vi "Fluke 28x Series Software Triggered Freqency Sweep.vi"() -> ()   [LabVIEW 2015]
doc: "This example shows how to configure a frequency sweep using a software trigger."
uses:
  <instrlib>/Fluke 28x Series/Fluke 28x Series.lvlib
panel:
  in  "Stop  Frequency  (1000.0 Hz)":dbl=1000.0 format="%#.6f"
  in  "Start Frequency (100.0 Hz)":dbl=100.0 format="%#.6g"
  in  "Sweep Time (1.00 s)":dbl=1.0 format="%#.6g"
  in  "Sweep Type (0: Continuous)":u16(ring) items=["Continuous", "Triggered", "Triggered, Hold/Reset"]
  in  "Amplitude (1.0 Vpp)":dbl=1.0
  in  "Waveform Function (0: Sine)":u16(ring) items=["Sine", "Square", "Triangle", "Cosine", "DC", "Positive Ramp", "Negative Ramp", "Haversine", "Havercosine", "Sine (x)/x"]
  in  "Channel (1)":u32(ring)=1 items=["1"=1, "2"=2, "3"=3, "4"=4]
  in  "VISA resource name":refnum<visa-resource-name>
  # "(c) 2009-2014 National Instruments.  ALL RIGHTS RESERVED."
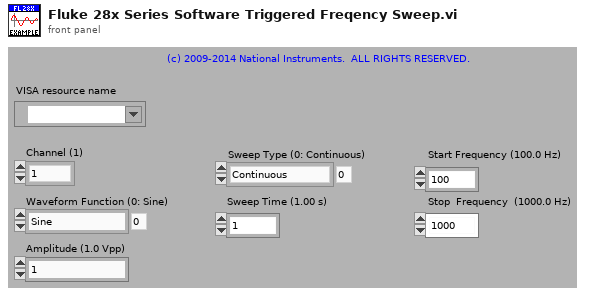
[diagram p1: front panel]
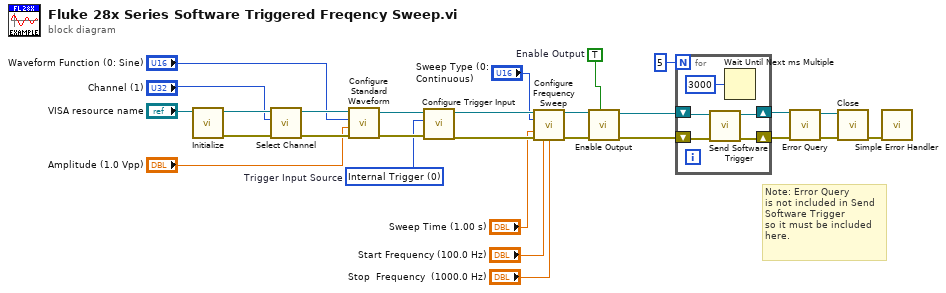
[diagram p0: block diagram]
diagram:
  w18 = u16 0 items=["Internal Trigger", "External Trigger", "Manual Trigger", "Channel Source"]  # Trigger Input Source
  w12 = TRUE  # Enable Output
  # "Note: Error Query\nis not included in Send\nSoftware Trigger\nso it must be included \nhere."
  n1 = call <instrlib>:"Initialize.vi"("VISA resource name"="VISA resource name") -> ("error out"=w26:errorcluster, "VISA resource name out"=w27:refnum<visa-resource-name>)  [unwired: 9 in]
  n2 = call <instrlib>:"Select Channel.vi"("error in (no error)"=w26, "Channel (1)"="Channel (1)", "VISA resource name"=w27) -> ("error out"=w24:errorcluster, "VISA resource name out"=w25:refnum<visa-resource-name>)  [unwired: 7 in]
  n3 = call <instrlib>:"Configure Standard Waveform.vi"("error in (no error)"=w24, "Amplitude (1.0 Vpp)"="Amplitude (1.0 Vpp)", "Waveform Function (0: Sine)"="Waveform Function (0: Sine)", "VISA resource name"=w25) -> ("error out"=w19:errorcluster, "VISA resource name out"=w20:refnum<visa-resource-name>)  [unwired: 6 in]
  n4 = call <instrlib>:"Configure Trigger Input.vi"("error in (no error)"=w19, "Trigger Input Source (0: Internal Trigger)"=w18, "VISA resource name"=w20) -> ("error out"=w16:errorcluster, "VISA resource name out"=w17:refnum<visa-resource-name>)  [unwired: 7 in]
  n5 = call <instrlib>:"Configure Frequency Sweep.vi"("VISA resource name"=w17, "Sweep Type (0: Continuous)"="Sweep Type (0: Continuous)", "Sweep Time (1.00 s)"="Sweep Time (1.00 s)", "error in (no error)"=w16, "Start Frequency (100.0 Hz)"="Start Frequency (100.0 Hz)", "Stop  Frequency  (1000.0 Hz)"="Stop  Frequency  (1000.0 Hz)") -> ("VISA resource name out"=w22:refnum<visa-resource-name>, "error out"=w21:errorcluster)  [unwired: 8 in]
  n6 = call <instrlib>:"Enable Output.vi"("Enable Output (T: Enable)"=w12, "error in (no error)"=w21, "VISA resource name"=w22) -> ("error out"=w14:errorcluster, "VISA resource name out"=w15:refnum<visa-resource-name>)  [unwired: 7 in]
  n7 = for {
    N: 5 -> [_]
    shift-right: [w32] -> w11
    shift-left: w15 -> [w33]
    shift-right: [w31] -> w10
    shift-left: w14 -> [w30]
    n8 = call <instrlib>:"Send Software Trigger.vi"("error in (no error)"=w30, "VISA resource name"=w33) -> ("error out"=w31:errorcluster, "VISA resource name out"=w32:refnum<visa-resource-name>)  [unwired: 8 in]
    n9 = Wait Until Next ms Multiple(millisecond multiple=u32 3000) -> ()  [unwired: 1 out]
  }
  n10 = call <instrlib>:"Error Query.vi"("error in (no error)"=w10, "VISA resource name"=w11) -> ("error out"=w8:errorcluster, "VISA resource name out"=w9:refnum<visa-resource-name>)  [unwired: 6 in, 2 out]
  n11 = call <instrlib>:"Close.vi"("error in (no error)"=w8, "VISA resource name"=w9) -> ("error out"=w23:errorcluster)  [unwired: 9 in]
  n12 = call <vilib>:"Simple Error Handler.vi"("error in (no error)"=w23) -> ()  [unwired: 4 in, 5 out]
